vi "dfd_SCL_ASymFIRm_Even_Cu.vi"(9 "global reset":bool, 10 "output valid":bool, 11 "index":i16) -> (1 "control info":T1)   [LabVIEW 2017]
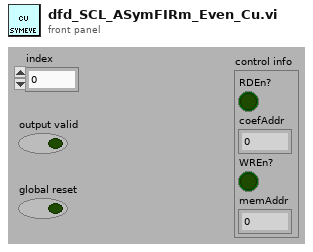
[diagram p1: front panel]
types:
  T1 = cluster{"RDEn?":bool, "coefAddr":u16, "WREn?":bool, "memAddr":u16}
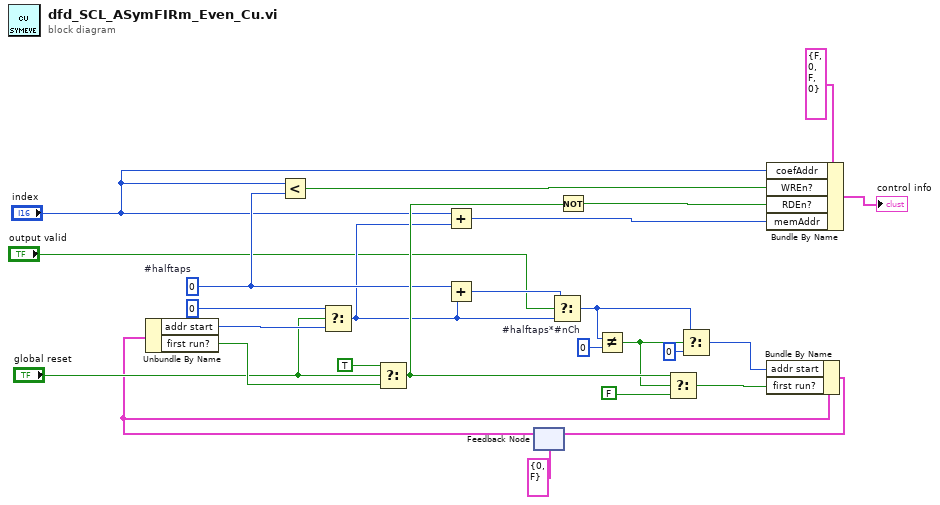
[diagram p0: block diagram]
diagram:
  w14 = u16 0  # #halftaps*#nCh
  w8 = i16 0  # #halftaps
  n1 = Less?(x="index", y=w8) -> (x < y?=w7:bool)
  n2 = feedback #1(cluster{"addr start":u16, "first run?":bool} {"addr start"=0, "first run?"=FALSE} ("states")) -> (w1:cluster{"addr start":u16, "first run?":bool})
  n3 = Unbundle By Name(w1) -> ("addr start"=w25:u16, "first run?"=w26:bool)
  n4 = Select(t=u16 0, s="global reset", f=w25) -> (s? t:f=w5:u16)
  n5 = Select(t=TRUE, s="global reset", f=w26) -> (s? t:f=w22:bool)
  n6 = Add(x="index", y=w5) -> (x+y=w10:u16)
  n7 = Add(x=w8, y=w5) -> (x+y=w16:u16)
  n8 = Select(t=w16, s="output valid", f=w5) -> (s? t:f=w17:u16)
  n9 = Not(x=w22) -> (.not. x?=w9:bool)
  n10 = Not Equal?(x=w17, y=w14) -> (x != y?=w19:bool)
  n11 = Select(t=w22, s=w19, f=FALSE ("t")) -> (s? t:f=w24:bool)
  n12 = Select(t=w17, s=w19, f=u16 0) -> (s? t:f=w23:u16)
  n13 = Bundle By Name(cluster=T1 {"RDEn?"=FALSE, "coefAddr"=0, "WREn?"=FALSE, "memAddr"=0} ("control info 2"), "coefAddr"="index", "WREn?"=w7, "RDEn?"=w9, "memAddr"=w10) -> (→"control info":T1)
  n14 = Bundle By Name(cluster=w1, "addr start"=w23, "first run?"=w24) -> (w4:cluster{"addr start":u16, "first run?":bool})
  n15 = feedback-in #1(w4) -> ()
